vi "Start Module.vi"(8 "error in (no error)":errorcluster, 10 "Cfg File Path":path, 11 "EventLog.lvclass":refnum<class "EventLog.lvclass">) -> (0 "error out":errorcluster, 1 "Wait for Event Sync?":bool, 2 "Tool Module Broadcast Events":T1)   [LabVIEW 2015, in "Tool Module.lvlib"]
doc: "Launches the Module Main.vi.\n_____\nBased on Delacor QMH Project Template 2.1.0.2."
uses:
  Tool Module.lvlib
  Broadcast Events--cluster.ctl
  Did Init Argument--cluster.ctl
  Status Updated Argument--cluster.ctl
  Error Reported Argument--cluster.ctl
  Stop Argument--cluster.ctl
  Get Module Execution Status Argument--cluster.ctl
  Send Status Argument--cluster.ctl
  Support/_STATUS Typedef--cluster.ctl
  Trigger Argument--cluster.ctl
  Connected Argument--cluster.ctl
  Read from File Rtn Argument--cluster.ctl
  Device Temperature Argument--cluster.ctl
  Tool Typedefs/_Temperature All Arrays--typedef.ctl
  Time Expired Argument--cluster.ctl
  QC-X App/Libraries/Event Logger Library/Event Log/EventLog.lvclass
  <vilib>/Delacor/Delacor QMH/Libraries/Module Admin_class/Delacor_lib_QMH_Module Admin.lvclass
  <vilib>/Delacor/Delacor QMH/Libraries/Module Admin_class/Delacor_lib_QMH_Module Admin.lvclass/Delacor_lib_QMH_Module Admin.ctl
  <vilib>/Delacor/Delacor QMH/Libraries/Module Admin_class/Delacor_lib_QMH_Set External Launch.vi
  <vilib>/Utility/error.llb/Error Cluster From Error Code.vi
  <vilib>/ErrorRing/Error Ring.xnode
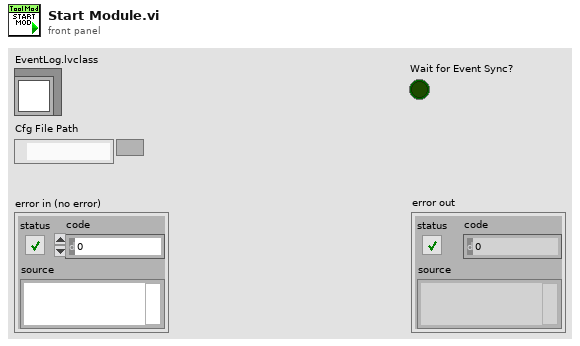
[diagram p1: front panel]
types:
  T1 = typedef "Tool Module.lvlib/Broadcast Events--cluster.ctl" = cluster{"Module Did Init":refnum<user-event>, "Status Updated":refnum<user-event>, "Error Reported":refnum<user-event>, "Module Did Stop":refnum<user-event>, "Update Module Execution Status":refnum<user-event>, "Send Status":refnum<user-event>, "Trigger":refnum<user-event>, "Connected":refnum<user-event>, "Read from File Rtn":refnum<user-event>, "Device Temperature":refnum<user-event>, "Time Expired":refnum<user-event>}
  T2 = enum32{"Bad", "Idle", "Run top level", "Running"}
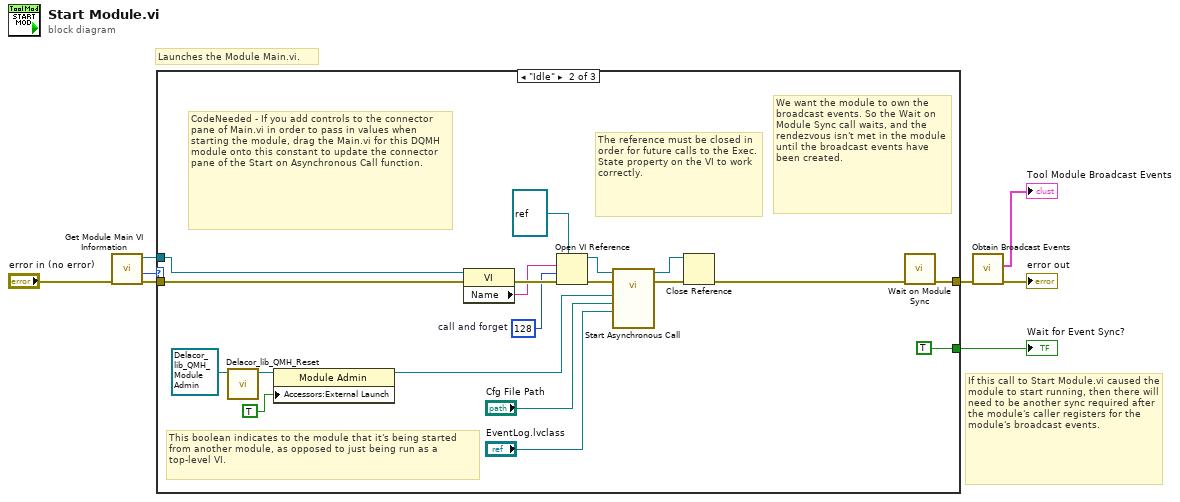
[diagram p0: block diagram]
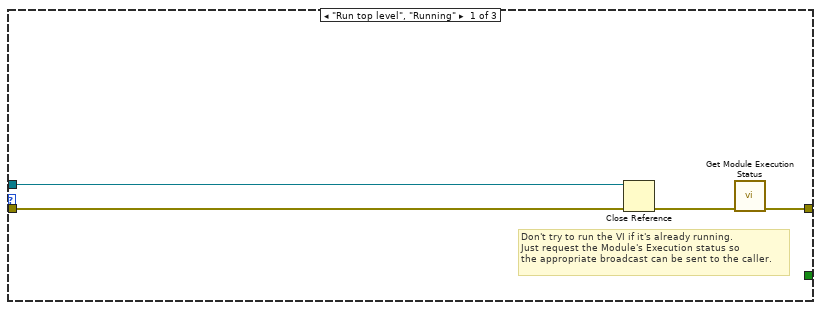
[diagram p2: hidden frame]
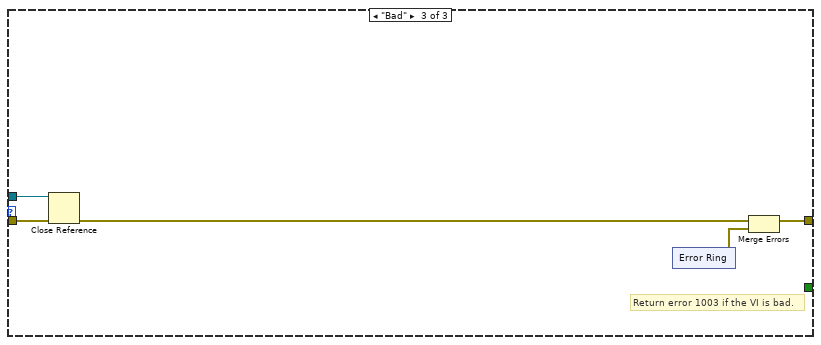
[diagram p3: hidden frame]
diagram:
  # "If this call to Start Module.vi caused the module to start running, then there will need to be another sync required after the module's caller registers for the module's broadcast events."
  # "Launches the Module Main.vi."
  n1 = call "Get Module Main VI Information.vi"("error in (no error)"="error in (no error)") -> ("error out"=w7:errorcluster, "Execution State"=w2:T2, "Module Main VI"=w6:refnum<vi>)  [unwired: 7 in, 1 out]
  n2 = case shown="\"Idle\"" w2 {
    tunnel: w7 -> [w12 w17 w36]
    tunnel: w6 -> [w11 w18 w35]
    tunnel: [w9 w30 w33] -> w5
    tunnel: [_ TRUE _] -> w3
    frame "Run top level", "Running" {
      # "Don't try to run the VI if it's already running.\nJust request the Module's Execution status so\nthe appropriate broadcast can be sent to the caller."
      n3 = Close Reference(reference=w11, error in (no error)=w12) -> (error out=w10:errorcluster)
      n4 = call "Get Module Execution Status.vi"("error in (no error)"=w10) -> ("error out"=w9:errorcluster)  [unwired: 10 in]
    }
    frame "Idle" {
      w19 = 128  # call and forget
      # "CodeNeeded - If you add controls to the connector pane of Main.vi in order to pass in values when starting the module, drag the Main.vi for this DQMH module onto this constant to update the connector pane of the Start on Asynchronous Call function."
      # "The reference must be closed in order for future calls to the Exec.State property on the VI to work correctly."
      # "We want the module to own the broadcast events. So the Wait on Module Sync call waits, and the rendezvous isn't met in the module until the broadcast events have been created."
      # "This boolean indicates to the module that it's being started from another module, as opposed to just being run as a top-level VI."
      n5 = call-dynamic "Delacor_lib_QMH_Reset.vi"("Mod Admin in"=refnum<class "Delacor_lib_QMH_Module Admin.lvclass"> refnum) -> ("Mod Admin out"=w28:refnum<class "Delacor_lib_QMH_Module Admin.lvclass">)  [unwired: 9 in, 1 out]
      n6 = property class="Module Admin"(reference=w28, "Accessors:External Launch"=TRUE) -> (reference out=w15:refnum<class "Delacor_lib_QMH_Module Admin.lvclass">)  [unwired: 1 in, 1 out]
      n7 = property class="VI"(reference=w18, error in=w17) -> (error out=w31:errorcluster, "Name"=w24:string)  [unwired: 1 out]
      n8 = Open VI Reference(type specifier VI Refnum (for type only)=refnum<vi> refnum, vi path=w24, options=w19, error in (no error)=w31) -> (vi reference=w21:refnum<vi>, error out=w20:errorcluster)  [unwired: 2 in]
      n9 = call-by-ref "Start Asynchronous Call"(reference=w21, error in=w20, "EventLog.lvclass"="EventLog.lvclass", "Cfg File Path"="Cfg File Path", "Module Admin"=w15) -> (reference out=w23:refnum<vi>, error out=w22:errorcluster)  [unwired: 9 in]
      n10 = Close Reference(reference=w23, error in (no error)=w22) -> (error out=w16:errorcluster)
      n11 = call "Wait on Module Sync.vi"("error in (no error)"=w16) -> ("error out"=w30:errorcluster)  [unwired: 10 in]
    }
    frame "Bad" {
      # "Return error 1003 if the VI is bad."
      n12 = Close Reference(reference=w35, error in (no error)=w36) -> (error out=w34:errorcluster)
      n13 = xnode "Error Ring"() -> ("error out"=w32:errorcluster)
      n14 = Merge Errors(w34, w32) -> (w33:errorcluster)
    }
  }
  "Wait for Event Sync?" <- w3
  n15 = call "Obtain Broadcast Events.vi"("error in (no error)"=w5) -> ("error out"=→"error out":errorcluster, "Tool Module Broadcast Events"=→"Tool Module Broadcast Events":T1)  [unwired: 9 in]
